vi "Remote_Request.vi"(7 "FIDs":u8[](array[numeric])=[6], 8 "error in (no error)":errorcluster, 9 "Retry interval (ms)":u32, 10 "Number of tries":u32, 11 "RREQ Packet":T2) -> (0 "error out":errorcluster, 1 "Processed Bytes":u8[][](array[numeric]), 2 "RREQ Param Out":T1, 3 "RREQ Packet Out":T2)   [LabVIEW 2017]
uses:
  Controls/Packet/Packet.ctl
  Controls/Packet/Packet_Direction.ctl
  Controls/Packet/Packet_Type.ctl
  Controls/Packet/Packet_Priority.ctl
  Controls/Control Packets/RREQ_Param.ctl
  <vilib>/Instr/_visa.llb/VISA Flush IO Buffer Mask.ctl
panel:
  out "Number of tries":i32
  out "Raw Bytes":u8[][](array[numeric])
  out "Current Frame Index":u8
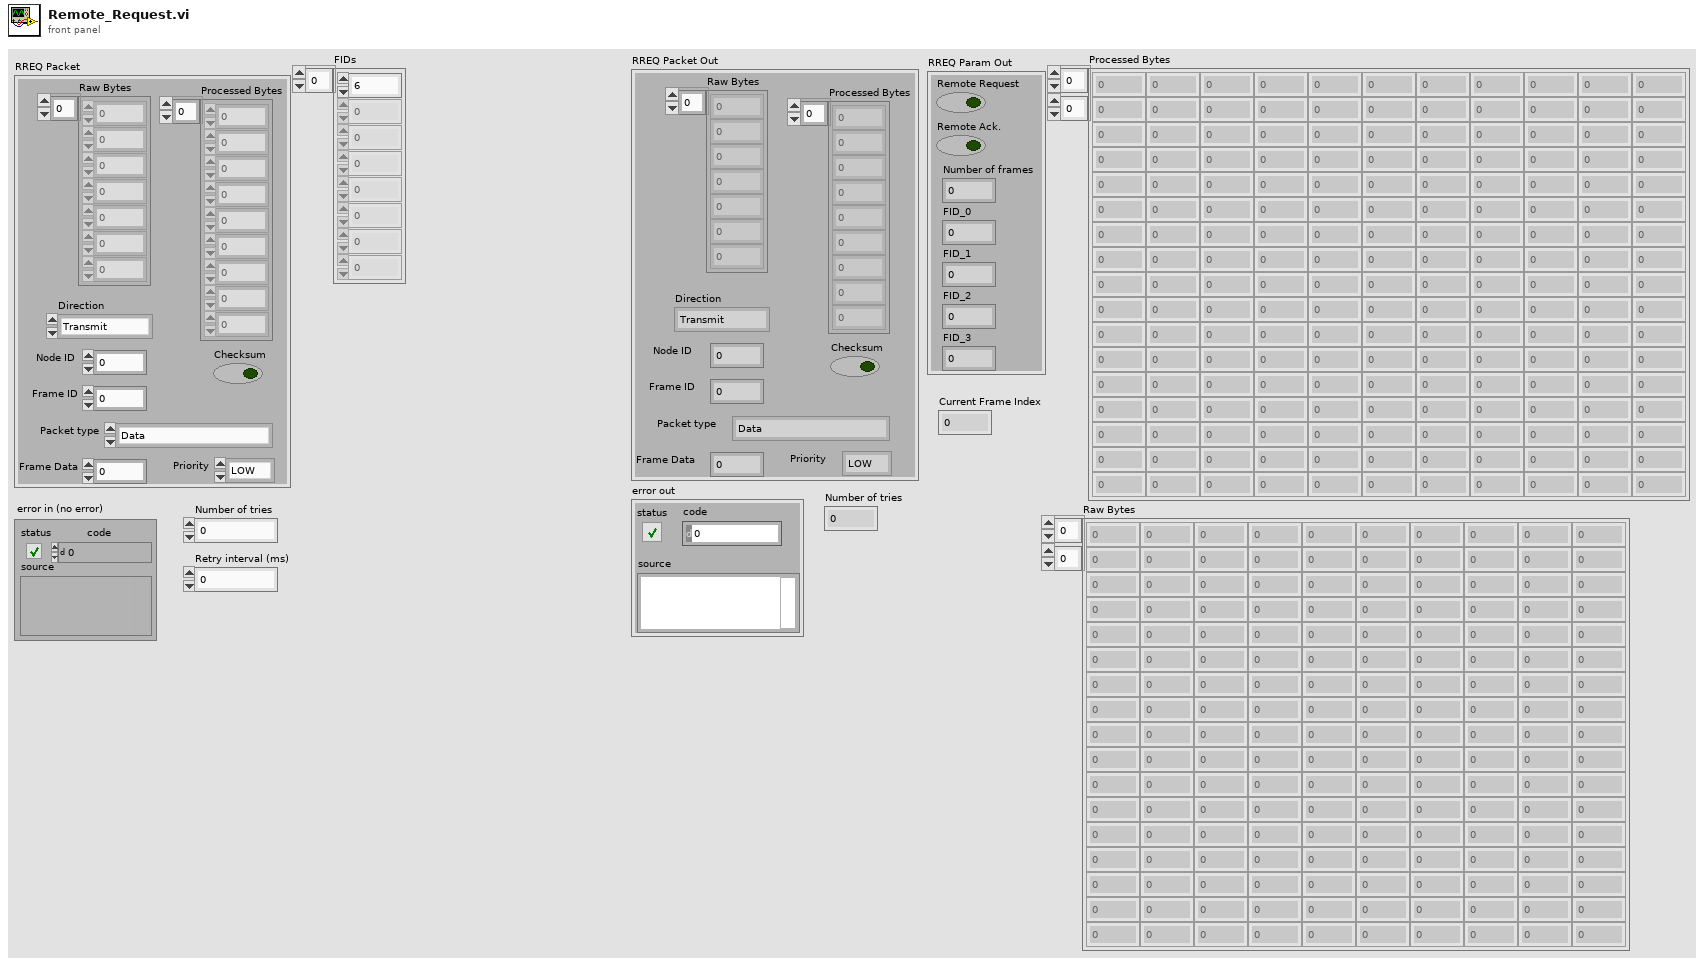
[diagram p1: front panel]
types:
  T1 = typedef "RREQ_Param.ctl" = cluster{"Remote Request":bool, "Remote Ack.":bool, "Number of frames":u8, "FID_0":u8, "FID_1":u8, "FID_2":u8, "FID_3":u8}
  T2 = typedef "Packet.ctl" = cluster{"Raw Bytes":u8[], "Checksum":bool, "Direction":T3, "Processed Bytes":u8[], "Node ID":u8, "Packet type":T4, "Frame Data":u32, "Priority":T5, "Frame ID":u8}
  T3 = typedef "Packet_Direction.ctl" = enum16{"Transmit", "Receive", "Bidirectional"}
  T4 = typedef "Packet_Type.ctl" = enum16{"Data", "Connection Management", "Remote Request", "Error/Status"}
  T5 = typedef "Packet_Priority.ctl" = enum16{"LOW", "HIGH"}
  T6 = typedef "VISA Flush IO Buffer Mask.ctl" = u16
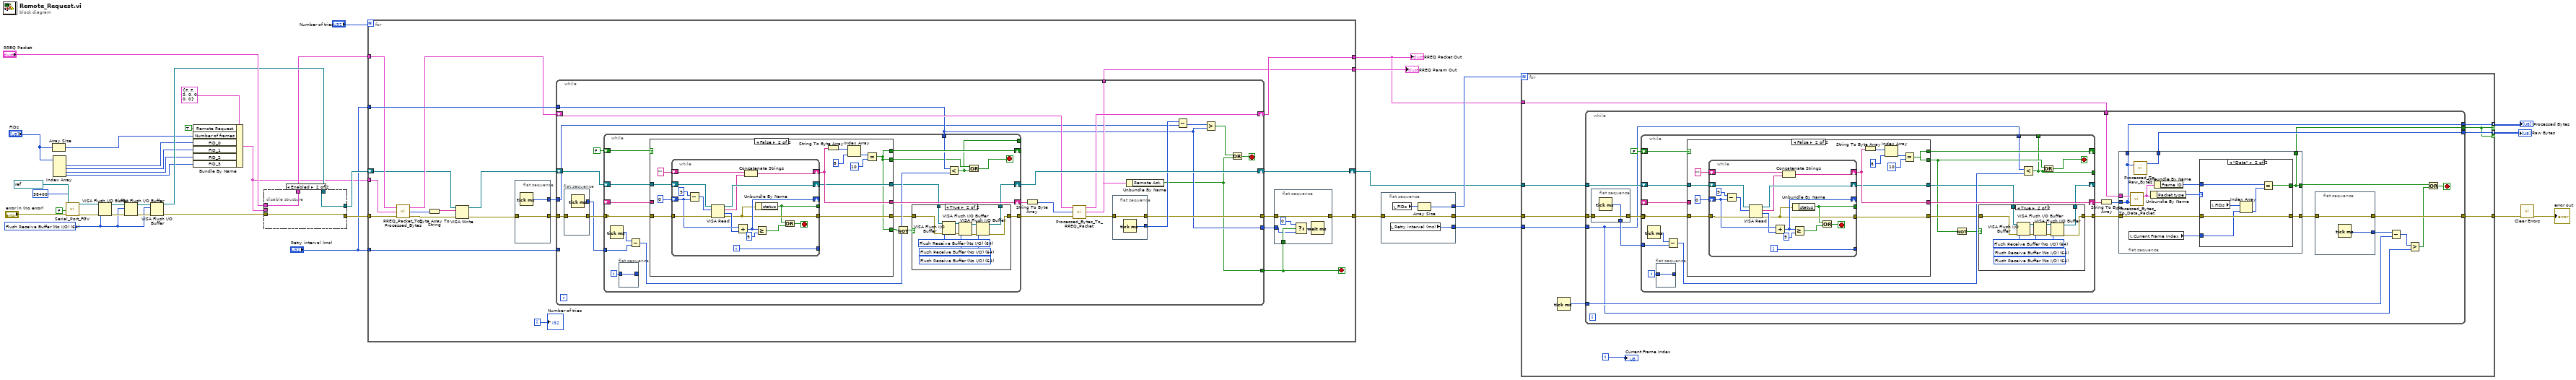
[diagram p0: block diagram]
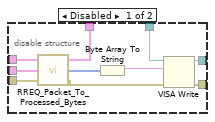
[diagram p2: hidden frame]
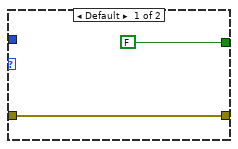
[diagram p3: hidden frame]
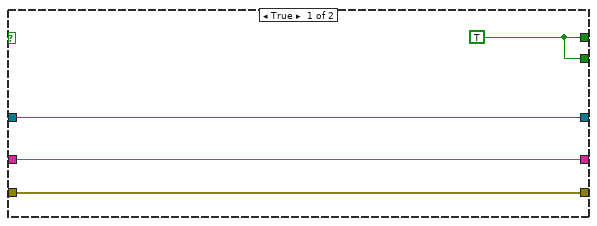
[diagram p5: hidden frame]
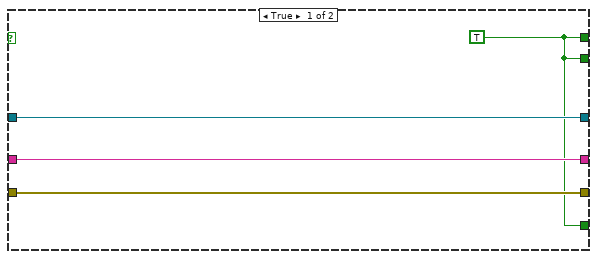
[diagram p7: hidden frame]
diagram:
  w31 = T6 64 items=["Flush Receive Buffer"=16, "Write Transmit Buffer to Device"=32, "Flush Receive Buffer (No I/O)"=64, "Flush Transmit Buffer"=128] ("Mask")
  n1 = Array Size(array="FIDs") -> (size(s)=w19:i32)
  n2 = Index Array(array="FIDs") -> (element #1=w17:u8, element #2=w16:u8, element #3=w15:u8, element #4=w14:u8)  [unwired: 4 in]
  n3 = call "Serial_Port_FGV.vi"("error in (no error)"="error in (no error)", "Initialize ?"=FALSE, "baud rate"=u32 38400, "COM Port In"=refnum<visa-resource-name> "COM17") -> ("error out"=w37:errorcluster, "COM Port out"=w36:refnum<visa-resource-name>)  [unwired: 6 in]
  n4 = VISA Flush I/O Buffer(VISA resource name=w36, mask (16)=w31, error in (no error)=w37) -> (VISA resource name out=w35:refnum<visa-resource-name>, error out=w34:errorcluster)
  n5 = VISA Flush I/O Buffer(VISA resource name=w35, mask (16)=w31, error in (no error)=w34) -> (VISA resource name out=w33:refnum<visa-resource-name>, error out=w32:errorcluster)
  n6 = VISA Flush I/O Buffer(VISA resource name=w33, mask (16)=w31, error in (no error)=w32) -> (VISA resource name out=w28:refnum<visa-resource-name>, error out=w30:errorcluster)
  n7 = Bundle By Name(cluster=T1 {"Remote Request"=FALSE, "Remote Ack."=FALSE, "Number of frames"=0, "FID_0"=0, "FID_1"=0, "FID_2"=0, "FID_3"=0} ("Cluster"), "Remote Request"=TRUE, "Number of frames"=w19, "FID_0"=w17, "FID_1"=w16, "FID_2"=w15, "FID_3"=w14) -> (w4:T1)
  n8 = disable-structure shown="Enabled" {
    disable-tunnel: w30 -> [w49 w50]
    disable-tunnel: "RREQ Packet" -> [w48 w51]
    disable-tunnel: w28 -> [w45 w52]
    disable-tunnel: [w43 w50] -> w27
    disable-tunnel: [w42 w52] -> w26
    disable-tunnel: [w41 w51] -> w23
    disable-tunnel: w4 -> [w40 _]
    frame Disabled {
      n9 = call "RREQ_Packet_To_Processed_Bytes.vi"("error in (no error)"=w49, "RREQ Param In"=w40, "RREQ Packet In"=w48) -> ("error out"=w46:errorcluster, "Processed Bytes"=w47:u8[], "RREQ Packet Out"=w41:T2)
      n10 = Byte Array To String(unsigned byte array=w47) -> (string=w44:string)
      n11 = VISA Write(VISA resource name=w45, write buffer=w44, error in (no error)=w46) -> (VISA resource name out=w42:refnum<visa-resource-name>, error out=w43:errorcluster)  [unwired: 1 out]
    }
    frame Enabled {
    }
  }
  n12 = for {
    N: "Number of tries" -> [_]
    tunnel: w27 -> [w63]
    shift-right: [w72] -> w5
    shift-left: w26 -> [w55]
    tunnel: "Retry interval (ms)" -> [w74]
    tunnel: "Retry interval (ms)" -> [w73]
    tunnel: w23 -> [w58]
    tunnel: [w71] -> w9
    tunnel: [w70] -> w22
    tunnel: [w68] -> w13
    tunnel: w4 -> [w62]
    i -> [w64]
    stop <- w65 stop-if-true
    n13 = call "RREQ_Packet_To_Processed_Bytes.vi"("error in (no error)"=w63, "RREQ Param In"=w62, "RREQ Packet In"=w58) -> ("error out"=w60:errorcluster, "Processed Bytes"=w59:u8[], "RREQ Packet Out"=w57:T2)
    n14 = Byte Array To String(unsigned byte array=w59) -> (string=w61:string)
    n15 = VISA Write(VISA resource name=w55, write buffer=w61, error in (no error)=w60) -> (VISA resource name out=w54:refnum<visa-resource-name>, error out=w56:errorcluster)  [unwired: 1 out]
    n16 = flat-sequence {
      tunnel: w56 -> [w76]
      tunnel: [w76] -> w66
      tunnel: [w75] -> w53
      frame #0 {
        n17 = Tick Count (ms)() -> (millisecond timer value=w75:u32)
      }
    }
    n18 = while {
      tunnel: w66 -> [w94]
      tunnel: w74 -> [_]
      tunnel: w73 -> [w87]
      tunnel: [w95] -> w70
      shift-right: [w101] -> w72
      shift-left: w54 -> [w102]
      shift-right: [w96] -> w71
      shift-left: w57 -> [w99]
      tunnel: [w88] -> w69
      tunnel: [w87] -> w67
      tunnel: [w86] -> w65
      tunnel: w53 -> [w83]
      stop <- w89 stop-if-true
      n19 = flat-sequence {
        tunnel: w94 -> [w106]
        tunnel: [w106] -> w93
        tunnel: [w105] -> w84
        frame #0 {
          n20 = Tick Count (ms)() -> (millisecond timer value=w105:u32)
        }
      }
      n21 = while {
        tunnel: w93 -> [w121]
        shift-right: [w124] -> _
        shift-left: FALSE -> [w125]
        tunnel: [w115] -> w100
        shift-right: [w123] -> w98
        shift-left: _ -> [w122]
        shift-right: [w113] -> w101
        shift-left: w102 -> [w126]
        tunnel: [w121] -> _
        tunnel: w84 -> [w119]
        tunnel: w87 -> [w117]
        tunnel: [w107] -> _
        i -> [w112]
        stop <- w111 stop-if-true
        n22 = Tick Count (ms)() -> (millisecond timer value=w120:u32)
        n23 = flat-sequence {
          tunnel: w112 -> [w127]
          tunnel: [w127] -> _
          frame #0 {
          }
        }
        n24 = Subtract(x=w120, y=w119) -> (x-y=w118:u32)
        n25 = case shown="False" w125 {
          tunnel: w121 -> [w144 w156]
          tunnel: w126 -> [w142 w154]
          tunnel: [w141 w145] -> w110
          tunnel: [w141 w145] -> w124
          tunnel: [w144 w148] -> w116
          tunnel: [w143 w147] -> w123
          tunnel: w122 -> [w143 _]
          tunnel: [w142 w146] -> w114
          tunnel: [w141 w145] -> w109
          frame True {
            w141 = TRUE
          }
          frame False {
            n26 = while {
              tunnel: w156 -> [w173]
              shift-right: [w163] -> _
              shift-left: 0 -> [w166]
              shift-right: [w169] -> w146
              shift-left: w154 -> [w170]
              shift-right: [w162] -> w147
              shift-left: "" -> [w168]
              tunnel: [w160] -> w148
              tunnel: [w161] -> _
              tunnel: [w157] -> _
              i -> [w161]
              stop <- w159 stop-if-true
              n27 = Subtract(x=9, y=w166) -> (x-y=w171:u32)
              n28 = VISA Read(VISA resource name=w170, byte count=w171, error in (no error)=w173) -> (VISA resource name out=w169:refnum<visa-resource-name>, read buffer=w167:string, return count=w165:u32, error out=w160:errorcluster)
              n29 = Add(x=w166, y=w165) -> (x+y=w163:u32)
              n30 = Concatenate Strings(w168, w167) -> (w162:string)
              n31 = Unbundle By Name(w160) -> ("status"=w157:bool)
              n32 = Greater Or Equal?(x=w163, y=u32 9) -> (x >= y?=w158:bool)
              n33 = Or(x=w157, y=w158) -> (x .or. y?=w159:bool)
            }
            n34 = String To Byte Array(string=w147) -> (unsigned byte array=w152:u8[])
            n35 = Index Array(array=w152, index=8) -> (element=w150:u8)
            n36 = Equal?(x=w150, y=u8 10) -> (x = y?=w145:bool)
          }
        }
        n37 = Not(x=w109) -> (.not. x?=w108:bool)
        n38 = case shown="True" w108 {
          tunnel: w116 -> [w129 w140]
          tunnel: [w129 w137] -> w115
          tunnel: w114 -> [w128 w136]
          tunnel: [w128 w133] -> w113
          frame False {
          }
          frame True {
            w130 = T6 64 items=["Flush Receive Buffer"=16, "Write Transmit Buffer to Device"=32, "Flush Receive Buffer (No I/O)"=64, "Flush Transmit Buffer"=128] ("Mask")
            w131 = T6 64 items=["Flush Receive Buffer"=16, "Write Transmit Buffer to Device"=32, "Flush Receive Buffer (No I/O)"=64, "Flush Transmit Buffer"=128] ("Mask")
            w132 = T6 64 items=["Flush Receive Buffer"=16, "Write Transmit Buffer to Device"=32, "Flush Receive Buffer (No I/O)"=64, "Flush Transmit Buffer"=128] ("Mask")
            n39 = VISA Flush I/O Buffer(VISA resource name=w136, mask (16)=w132, error in (no error)=w140) -> (VISA resource name out=w135:refnum<visa-resource-name>, error out=w139:errorcluster)
            n40 = VISA Flush I/O Buffer(VISA resource name=w135, mask (16)=w131, error in (no error)=w139) -> (VISA resource name out=w134:refnum<visa-resource-name>, error out=w138:errorcluster)
            n41 = VISA Flush I/O Buffer(VISA resource name=w134, mask (16)=w130, error in (no error)=w138) -> (VISA resource name out=w133:refnum<visa-resource-name>, error out=w137:errorcluster)
          }
        }
        n42 = Less?(x=w117, y=w118) -> (x < y?=w107:bool)
        n43 = Or(x=w110, y=w107) -> (x .or. y?=w111:bool)
      }
      n44 = String To Byte Array(string=w98) -> (unsigned byte array=w97:u8[])
      n45 = call "Processed_Bytes_To_RREQ_Packet.vi"("error in (no error)"=w100, "Processed Bytes"=w97, "RREQ Packet In"=w99) -> ("error out"=w92:errorcluster, "RREQ Param"=w95:T1, "RREQ Packet Out"=w96:T2)
      n46 = flat-sequence {
        tunnel: w92 -> [w104]
        tunnel: [w104] -> w88
        tunnel: [w103] -> w91
        frame #0 {
          n47 = Tick Count (ms)() -> (millisecond timer value=w103:u32)
        }
      }
      n48 = Unbundle By Name(w95) -> ("Remote Ack."=w86:bool)
      n49 = Subtract(x=w91, y=w83) -> (x-y=w90:u32)
      n50 = Greater?(x=w90, y=w87) -> (0:w82:bool)
      n51 = Or(x=w82, y=w86) -> (x .or. y?=w89:bool)
    }
    n52 = flat-sequence {
      tunnel: w69 -> [w81]
      tunnel: [w81] -> w68
      tunnel: w67 -> [w78]
      tunnel: w65 -> [w79]
      frame #0 {
        n53 = Select(t=u32 0, s=w79, f=w78) -> (s? t:f=w80:u32)
        n54 = Wait (ms)(milliseconds to wait=w80) -> ()  [unwired: 1 out]
      }
    }
    "Number of tries" <- w64
  }
  "RREQ Packet Out" <- w9
  "RREQ Param Out" <- w22
  n55 = flat-sequence {
    tunnel: w13 -> [w177]
    tunnel: [w177] -> w12
    tunnel: [w176] -> w11
    tunnel: [w174] -> w10
    frame #0 {
      n56 = local read "Retry interval (ms)"() -> (w176:u32)
      n57 = local read "FIDs"() -> (w175:u8[])
      n58 = Array Size(array=w175) -> (size(s)=w174:i32)
    }
  }
  n59 = for {
    N: w10 -> [_]
    tunnel: w5 -> [w187]
    tunnel: w12 -> [w186]
    tunnel: w11 -> [w185]
    tunnel: w9 -> [w184]
    tunnel: [w182] -> w8
    tunnel: [w181] -> w7 mode=indexing if=w179
    tunnel: [w180] -> w6 mode=indexing if=w179
    i -> [w183]
    n60 = Tick Count (ms)() -> (millisecond timer value=w178:u32)
    n61 = while {
      tunnel: w187 -> [w207]
      tunnel: w186 -> [w197]
      tunnel: w185 -> [w189]
      tunnel: w184 -> [w203]
      tunnel: [w193] -> w182
      tunnel: [w202] -> w181
      tunnel: [w201] -> w180
      tunnel: [w200] -> w179
      tunnel: w178 -> [w191]
      stop <- w199 stop-if-true
      n62 = flat-sequence {
        tunnel: w197 -> [w212]
        tunnel: [w212] -> w196
        tunnel: [w211] -> w195
        frame #0 {
          n63 = Tick Count (ms)() -> (millisecond timer value=w211:u32)
        }
      }
      n64 = while {
        tunnel: w196 -> [w244]
        shift-right: [w247] -> _
        shift-left: FALSE -> [w248]
        tunnel: [w239] -> w206
        shift-right: [w246] -> w205
        shift-left: _ -> [w245]
        shift-right: [w237] -> _
        shift-left: w207 -> [w249]
        tunnel: [w244] -> _
        tunnel: w189 -> [w241]
        tunnel: w195 -> [w235]
        tunnel: [w231] -> _
        tunnel: [w231] -> _
        i -> [w236]
        stop <- w232 stop-if-true
        n65 = Tick Count (ms)() -> (millisecond timer value=w243:u32)
        n66 = flat-sequence {
          tunnel: w236 -> [w250]
          tunnel: [w250] -> _
          frame #0 {
          }
        }
        n67 = Subtract(x=w243, y=w235) -> (x-y=w242:u32)
        n68 = case shown="False" w248 {
          tunnel: w244 -> [w266 w279]
          tunnel: w249 -> [w264 w277]
          tunnel: [w267 w271] -> w234
          tunnel: [w267 w271] -> w247
          tunnel: [w266 w270] -> w240
          tunnel: [w265 w269] -> w246
          tunnel: w245 -> [w265 _]
          tunnel: [w264 w268] -> w238
          frame True {
            w267 = TRUE
          }
          frame False {
            n69 = while {
              tunnel: w279 -> [w296]
              shift-right: [w286] -> _
              shift-left: 0 -> [w289]
              shift-right: [w292] -> w268
              shift-left: w277 -> [w293]
              shift-right: [w285] -> w269
              shift-left: "" -> [w291]
              tunnel: [w283] -> w270
              tunnel: [w284] -> _
              tunnel: [w280] -> _
              i -> [w284]
              stop <- w282 stop-if-true
              n70 = Subtract(x=9, y=w289) -> (x-y=w294:u32)
              n71 = VISA Read(VISA resource name=w293, byte count=w294, error in (no error)=w296) -> (VISA resource name out=w292:refnum<visa-resource-name>, read buffer=w290:string, return count=w288:u32, error out=w283:errorcluster)
              n72 = Add(x=w289, y=w288) -> (x+y=w286:u32)
              n73 = Concatenate Strings(w291, w290) -> (w285:string)
              n74 = Unbundle By Name(w283) -> ("status"=w280:bool)
              n75 = Greater Or Equal?(x=w286, y=u32 9) -> (x >= y?=w281:bool)
              n76 = Or(x=w280, y=w281) -> (x .or. y?=w282:bool)
            }
            n77 = String To Byte Array(string=w269) -> (unsigned byte array=w275:u8[])
            n78 = Index Array(array=w275, index=8) -> (element=w273:u8)
            n79 = Equal?(x=w273, y=u8 10) -> (x = y?=w271:bool)
          }
        }
        n80 = Not(x=w234) -> (.not. x?=w233:bool)
        n81 = case shown="True" w233 {
          tunnel: w240 -> [w252 w263]
          tunnel: [w252 w260] -> w239
          tunnel: w238 -> [w251 w259]
          tunnel: [w251 w256] -> w237
          frame False {
          }
          frame True {
            w253 = T6 64 items=["Flush Receive Buffer"=16, "Write Transmit Buffer to Device"=32, "Flush Receive Buffer (No I/O)"=64, "Flush Transmit Buffer"=128] ("Mask")
            w254 = T6 64 items=["Flush Receive Buffer"=16, "Write Transmit Buffer to Device"=32, "Flush Receive Buffer (No I/O)"=64, "Flush Transmit Buffer"=128] ("Mask")
            w255 = T6 64 items=["Flush Receive Buffer"=16, "Write Transmit Buffer to Device"=32, "Flush Receive Buffer (No I/O)"=64, "Flush Transmit Buffer"=128] ("Mask")
            n82 = VISA Flush I/O Buffer(VISA resource name=w259, mask (16)=w255, error in (no error)=w263) -> (VISA resource name out=w258:refnum<visa-resource-name>, error out=w262:errorcluster)
            n83 = VISA Flush I/O Buffer(VISA resource name=w258, mask (16)=w254, error in (no error)=w262) -> (VISA resource name out=w257:refnum<visa-resource-name>, error out=w261:errorcluster)
            n84 = VISA Flush I/O Buffer(VISA resource name=w257, mask (16)=w253, error in (no error)=w261) -> (VISA resource name out=w256:refnum<visa-resource-name>, error out=w260:errorcluster)
          }
        }
        n85 = Less?(x=w241, y=w242) -> (x < y?=w231:bool)
        n86 = Or(x=w234, y=w231) -> (x .or. y?=w232:bool)
      }
      n87 = String To Byte Array(string=w205) -> (unsigned byte array=w204:u8[])
      n88 = flat-sequence {
        tunnel: w206 -> [w220]
        tunnel: w204 -> [w215]
        tunnel: w203 -> [w222]
        tunnel: [w219] -> w194
        tunnel: [w213] -> w198
        tunnel: [w215] -> w202
        tunnel: [w214] -> w201
        tunnel: [w213] -> w200
        frame #0 {
          n89 = local read "Current Frame Index"() -> (w216:u8)
          n90 = call "Processed_Bytes_To_Data_Packet.vi"("Processed Bytes"=w215, "Data Packet In"=w222) -> ("Data Packet Out"=w218:T2)  [unwired: 1 in]
          n91 = call "Processed_To_Raw_Bytes.vi"("Processed Bytes"=w215) -> ("Raw Bytes"=w214:u8[])  [unwired: 1 in, 4 out]
          n92 = Unbundle By Name(w218) -> ("Packet type"=w221:T4)
          n93 = Unbundle By Name(w218) -> ("Frame ID"=w217:u8)
          n94 = case shown="\"Data\"" w221 {
            tunnel: w220 -> [w224 w230]
            tunnel: [w224 w230] -> w219
            tunnel: [FALSE w225] -> w213
            tunnel: w217 -> [_ w226]
            tunnel: w216 -> [_ w228]
            frame Default {
            }
            frame "Data" {
              n95 = local read "FIDs"() -> (w229:u8[])
              n96 = Index Array(array=w229, index=w228) -> (element=w227:u8)
              n97 = Equal?(x=w226, y=w227) -> (x = y?=w225:bool)
            }
          }
        }
      }
      n98 = flat-sequence {
        tunnel: w194 -> [w210]
        tunnel: [w210] -> w193
        tunnel: [w209] -> w192
        frame #0 {
          n99 = Tick Count (ms)() -> (millisecond timer value=w209:u32)
        }
      }
      n100 = Subtract(x=w192, y=w191) -> (x-y=w190:u32)
      n101 = Greater?(x=w190, y=w189) -> (0:w188:bool)
      n102 = Or(x=w198, y=w188) -> (x .or. y?=w199:bool)
    }
    "Current Frame Index" <- w183
  }
  "Processed Bytes" <- w7
  "Raw Bytes" <- w6
  n103 = call <vilib>:"Clear Errors.vi"("error in (no error)"=w8) -> ("error out"=→"error out":errorcluster)  [unwired: 5 in, 1 out]
